vi "히로미사_TEST_2.vi"() -> ()   [LabVIEW 2023]
uses:
  <vilib>/Analysis/3filter.llb/Filter Passband Type.ctl
  <vilib>/Analysis/3filter.llb/Butterworth Filter (DBL).vi
  <vilib>/Analysis/2dsp.llb/1D Cross Correlation (DBL).vi
  <vilib>/Analysis/NI_AALBase.lvlib
  <vilib>/Analysis/NI_AALPro.lvlib
panel:
  in  "불리언":bool
  out "Phase_CR_CI_aTANT":waveform(dbl)(graph)
  out "Amplitude_CR_CI":waveform(dbl)(graph)
  out "Matched_CR_RESULT_Baseband":waveform(dbl)(graph)
  out "Matched_CI_RESULT_Baseband":waveform(dbl)(graph)
  out "Filter_Result_SIN":waveform(dbl)(graph)
  out "Filter_Result_COS":waveform(dbl)(graph)
  out "Local_Result_COS":waveform(dbl)(graph)
  out "Local_Result_SIN":waveform(dbl)(graph)
  out "Matched_CR_Result":waveform(dbl)(graph)
  out "Matched_CI_Result":waveform(dbl)(graph)
  out "RX SIG 그래프":waveform(dbl)(graph)
  in  "Delta_Phase":dbl=90.0 format="%#_13g"
  in  "INIT_phase":dbl=90.0 format="%#_13g"
  out "Mask CR 그래프":waveform(dbl)(graph)
  out "Mask CI 그래프":waveform(dbl)(graph)
  out "Cos_Q 결과 그래프":waveform(dbl)(graph)
  out "Sine_Q 결과 그래프":waveform(dbl)(graph)
  in  "Q":dbl=2.0 format="%#_13g"
  in  "위상":dbl format="%#_13g"
  in  "Fs":dbl=20000.0 format="%#_13g"
  in  "주파수":dbl=5.0 format="%#_13g"
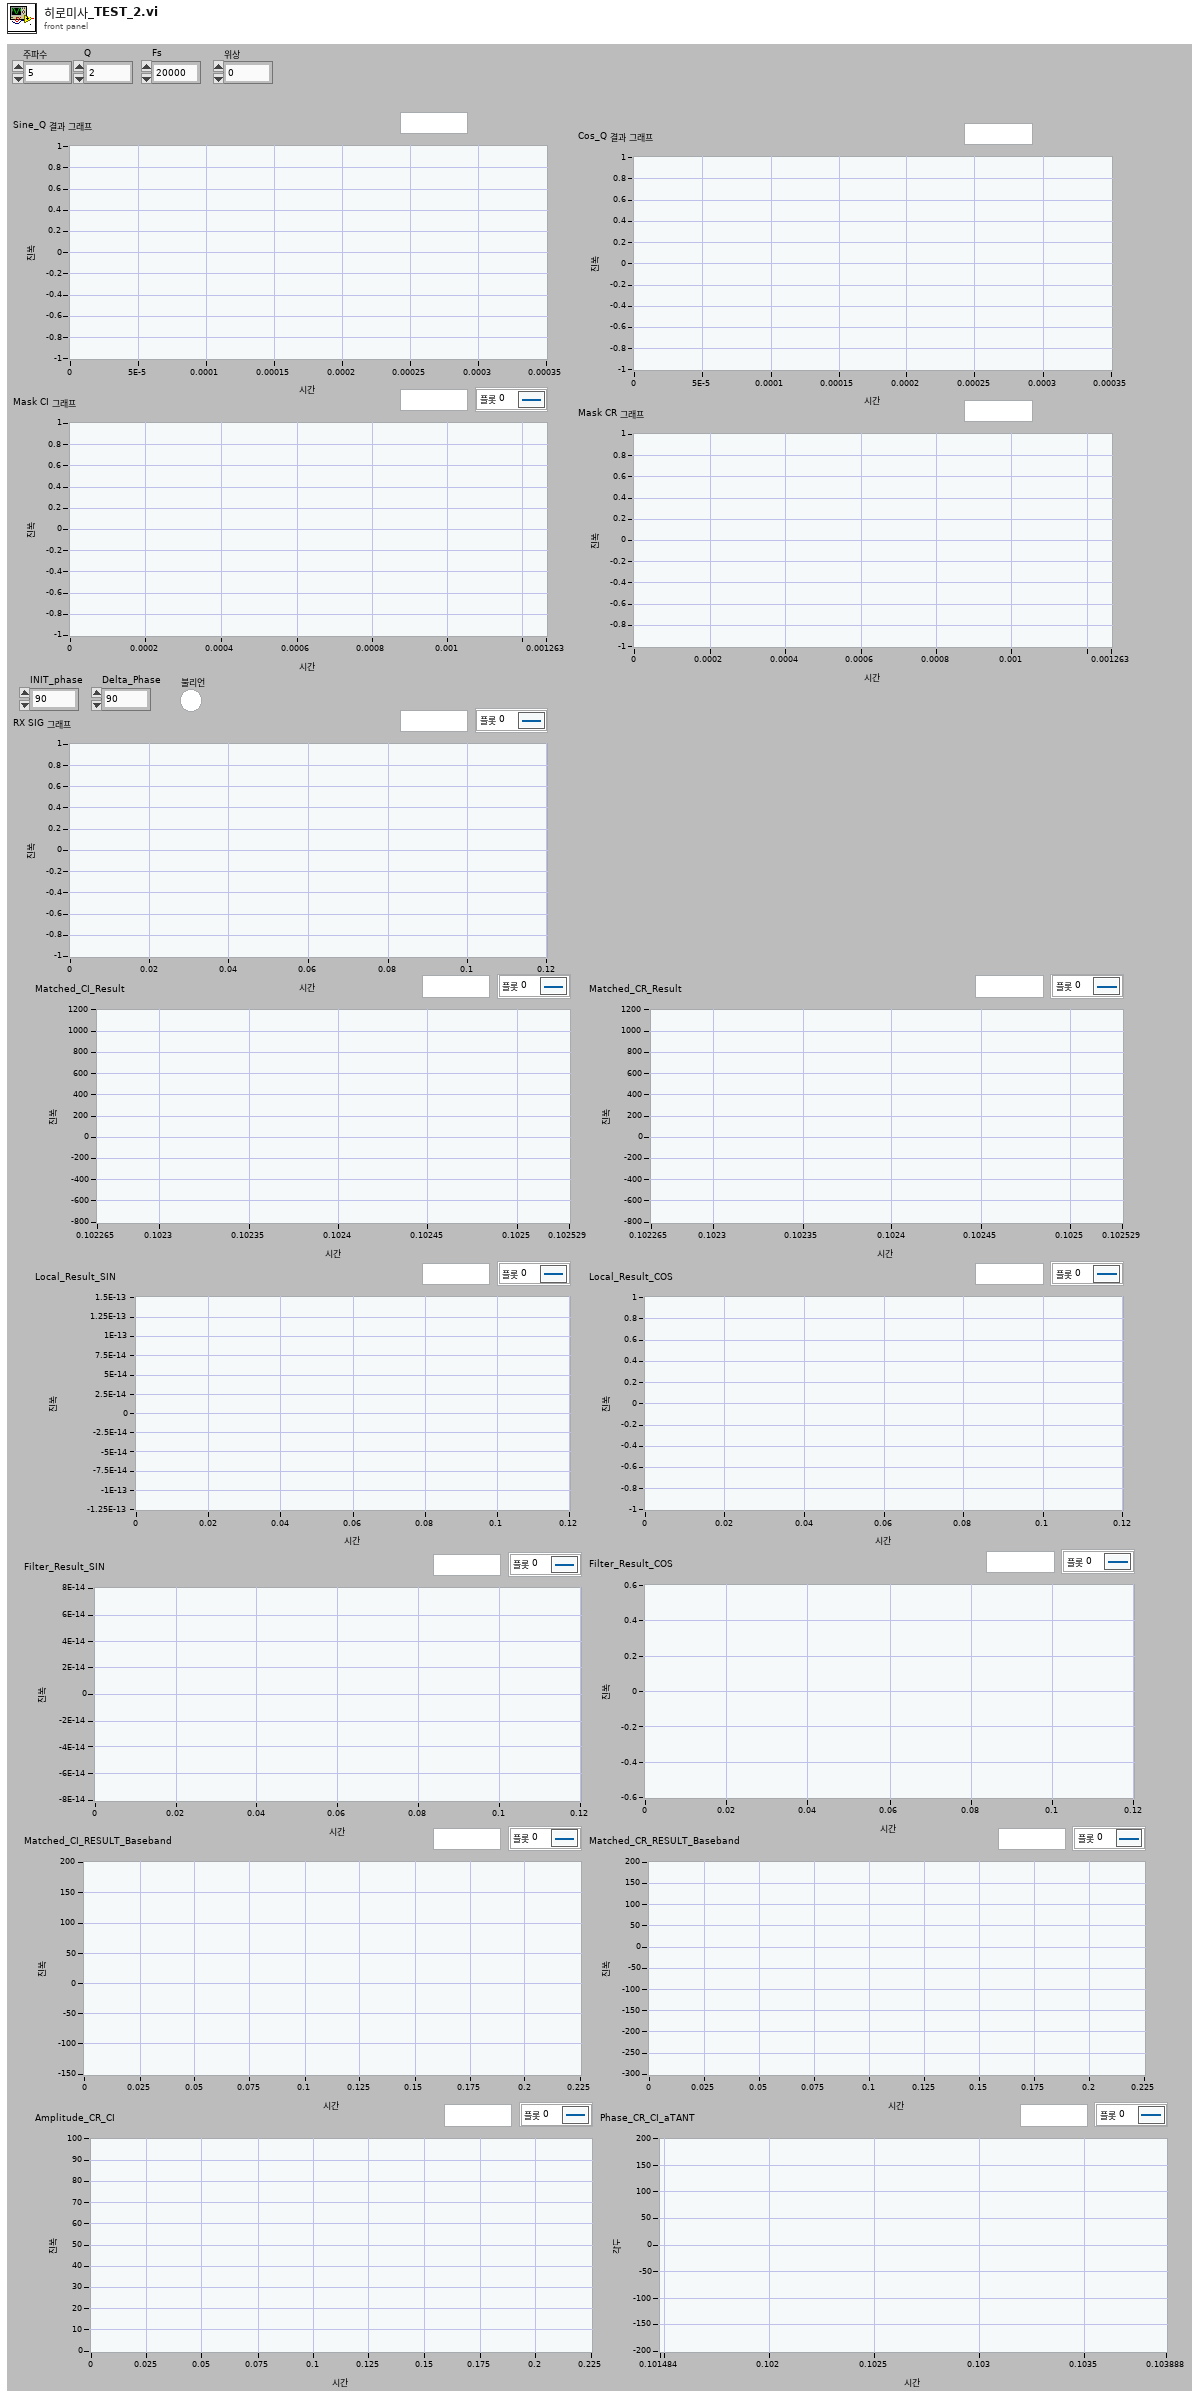
[diagram p1: front panel]
types:
  T1 = typedef "NI_AALBase.lvlib/Filter Passband Type.ctl" = enum32{"Lowpass", "Highpass", "Bandpass", "Bandstop"}
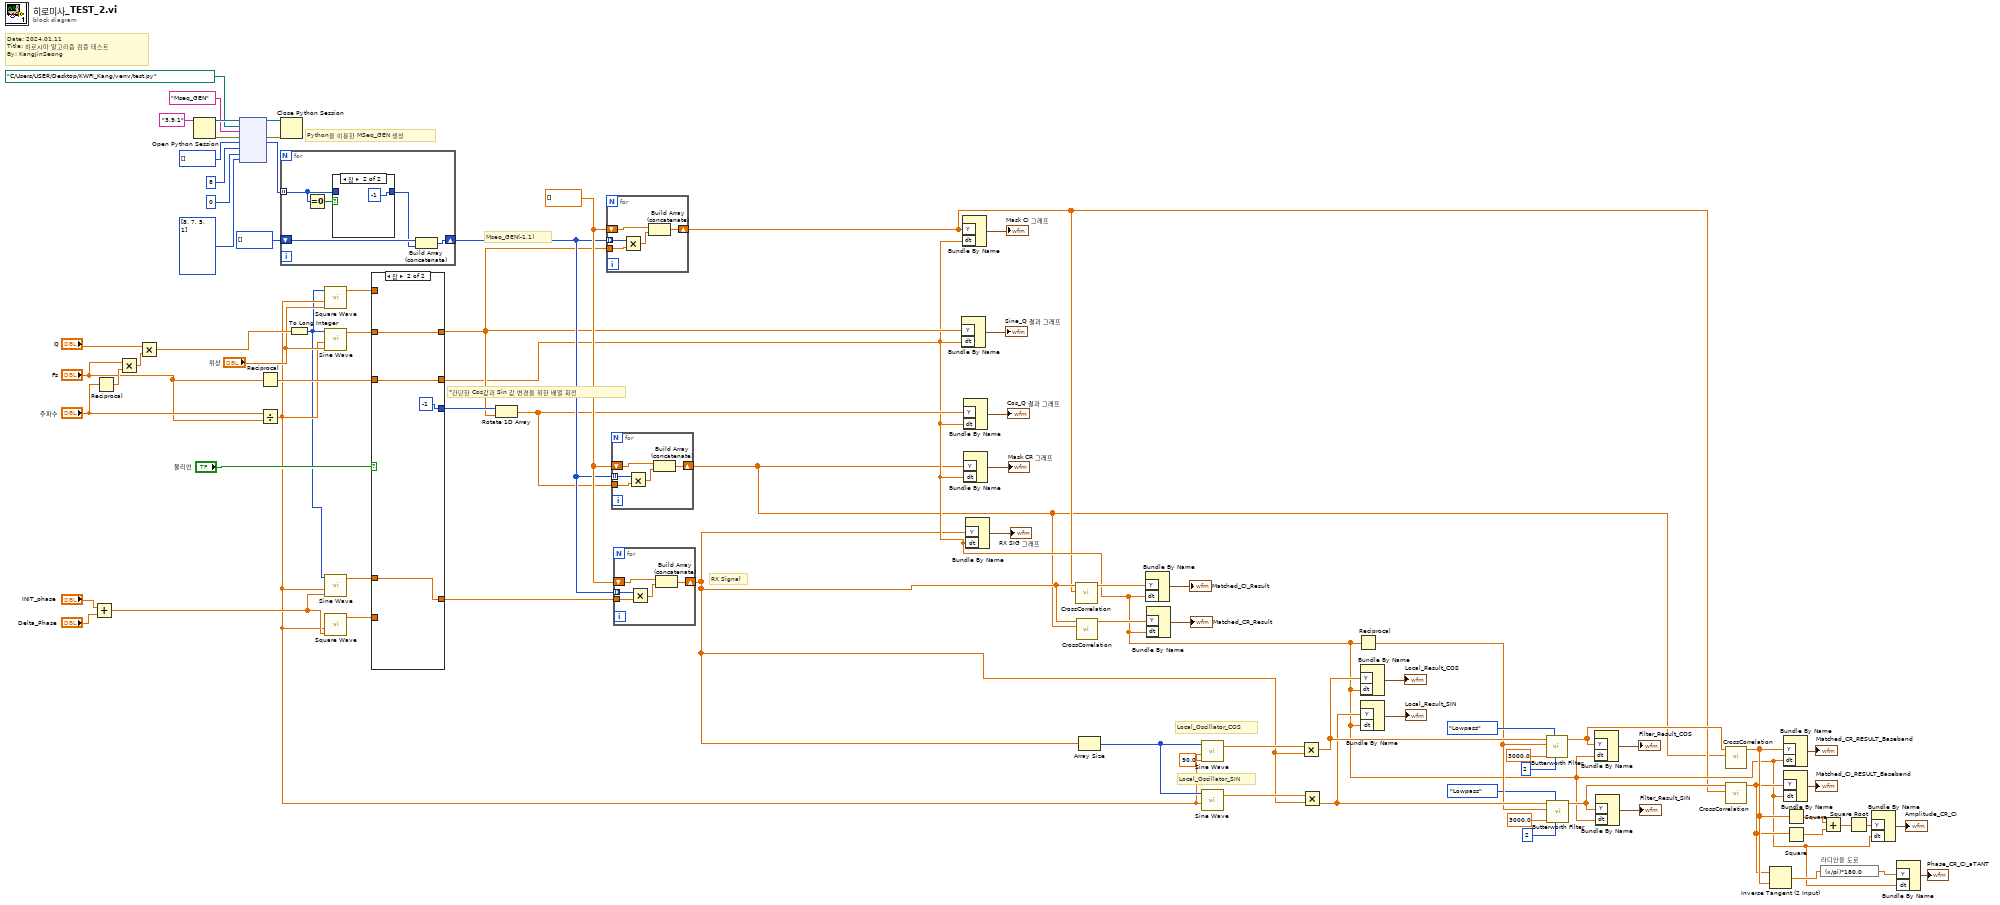
[diagram p0: block diagram]
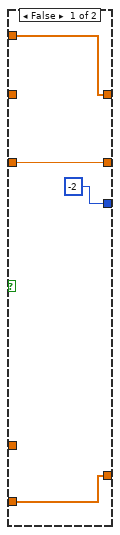
[diagram p2: hidden frame]
diagram:
  w52 = dbl[] []
  # "*간단한 Cos값과 Sin 값 변경을 위한 배열 회전"
  # "Mseq_GEN(-1,1)"
  # "Python을 이용한 MSeq_GEN 생성"
  # "Local_Oscillator_SIN"
  # "Local_Oscillator_COS"
  # "RX Signal"
  # "Date: 2024.01.11\nTitle: 히로시마 알고리즘 검증 테스트\nBy: KangJinSeong"
  n1 = Add(x="INIT_phase", y="Delta_Phase") -> (x+y=w18:dbl)
  n2 = Reciprocal(x="주파수") -> (1/x=w67:dbl)
  n3 = Multiply(x="Fs", y=w67) -> (x*y=w65:dbl)
  n4 = Multiply(x="Q", y=w65) -> (x*y=w63:dbl)
  n5 = Open Python Session(python version="3.9.1" ("Python 버전")) -> (session out=w80:refnum<k35>, error out=w79:errorcluster)  [unwired: 2 in]
  n6 = node(w80, path "C:/Users/USER/Desktop/KWFI_Kang/venv/test.py" ("Python 경로"), "Mseq_GEN" ("함수 이름"), w79, i32[] [], 8, 0, i32[] [8, 7, 5, 1]) -> (w77:refnum<k35>, w78:errorcluster, w69:i32[])  [unwired: 3 in, 2 out]
  n7 = Reciprocal(x="Fs") -> (1/x=w10:dbl)
  n8 = Divide(x="주파수", y="Fs") -> (x/y=w2:dbl)
  n9 = Close Python Session(session in=w77, error in=w78) -> ()  [unwired: 1 out]
  n10 = for {
    tunnel: w69 -> [w83] mode=indexing
    shift-right: [w82] -> w33
    shift-left: i32[] [] -> [w85]
    n11 = Equal To 0?(x=w83) -> (x = 0?=w86:bool)
    n12 = case shown="참" w86 {
      tunnel: [w87 -1] -> w84
      tunnel: w83 -> [w87 _]
      frame False {
      }
      frame True {
      }
    }
    n13 = Build Array (concatenate)(w85, w84) -> (w82:i32[])
  }
  n14 = To Long Integer(number=w63) -> (32bit integer=w1:i32)
  n15 = call <vilib>:"Square Wave.vi"("samples"=w1, "frequency"=w2, "phase in"="위상") -> ("square wave"=w16:dbl[])  [unwired: 3 in, 2 out]
  n16 = call <vilib>:"Sine Wave.vi"("samples"=w1, "frequency"=w2, "phase in"="위상") -> ("sine wave"=w15:dbl[])  [unwired: 2 in, 2 out]
  n17 = call <vilib>:"Sine Wave.vi"("samples"=w1, "frequency"=w2, "phase in"=w18) -> ("sine wave"=w14:dbl[])  [unwired: 2 in, 2 out]
  n18 = call <vilib>:"Square Wave.vi"("frequency"=w2, "phase in"=w18) -> ("square wave"=w12:dbl[])  [unwired: 4 in, 2 out]
  n19 = case shown="참" "불리언" {
    tunnel: w16 -> [w92 _]
    tunnel: w15 -> [_ w96]
    tunnel: [w92 w96] -> w9
    tunnel: w14 -> [_ w95]
    tunnel: [w91 w95] -> w13
    tunnel: w12 -> [w91 _]
    tunnel: [-2 ("n") -1 ("n")] -> w11
    tunnel: w10 -> [w89 w93]
    tunnel: [w89 w93] -> w7
    frame False {
    }
    frame True {
    }
  }
  n20 = Rotate 1D Array(1:w9, 2:w11) -> (0:w8:dbl[])
  n21 = for {
    tunnel: w9 -> [w100]
    tunnel: w33 -> [w101] mode=indexing
    shift-right: [w97] -> w5
    shift-left: w52 -> [w99]
    n22 = Multiply(x=w101, y=w100) -> (x*y=w98:dbl[])
    n23 = Build Array (concatenate)(w99, w98) -> (w97:dbl[])
  }
  n24 = for {
    tunnel: w8 -> [w105]
    tunnel: w33 -> [w106] mode=indexing
    shift-right: [w102] -> w4
    shift-left: w52 -> [w104]
    n25 = Multiply(x=w106, y=w105) -> (x*y=w103:dbl[])
    n26 = Build Array (concatenate)(w104, w103) -> (w102:dbl[])
  }
  n27 = for {
    tunnel: w33 -> [w111] mode=indexing
    shift-right: [w108] -> w6
    shift-left: w52 -> [w110]
    tunnel: w13 -> [w107]
    n28 = Multiply(x=w111, y=w107) -> (x*y=w109:dbl[])
    n29 = Build Array (concatenate)(w110, w109) -> (w108:dbl[])
  }
  n30 = Bundle By Name("Y"=w9, "dt"=w7) -> (→"Sine_Q 결과 그래프":waveform(dbl))  [unwired: 1 in]
  n31 = Bundle By Name("Y"=w5, "dt"=w7) -> (→"Mask CI 그래프":waveform(dbl))  [unwired: 1 in]
  n32 = Bundle By Name("Y"=w8, "dt"=w7) -> (→"Cos_Q 결과 그래프":waveform(dbl))  [unwired: 1 in]
  n33 = Bundle By Name("Y"=w4, "dt"=w7) -> (→"Mask CR 그래프":waveform(dbl))  [unwired: 1 in]
  n34 = Bundle By Name("Y"=w6, "dt"=w7) -> (→"RX SIG 그래프":waveform(dbl))  [unwired: 1 in]
  n35 = call-poly <vilib>:"CrossCorrelation.vi"("Y"=w5, "X"=w6) -> ("Rxy"=w56:dbl[])  [unwired: 8 in, 1 out]
  n36 = call-poly <vilib>:"CrossCorrelation.vi"("Y"=w4, "X"=w6) -> ("Rxy"=w53:dbl[])  [unwired: 8 in, 1 out]
  n37 = Array Size(array=w6) -> (size(s)=w50:i32)
  n38 = Bundle By Name("Y"=w56, "dt"=w7) -> (→"Matched_CI_Result":waveform(dbl))  [unwired: 1 in]
  n39 = Bundle By Name("Y"=w53, "dt"=w7) -> (→"Matched_CR_Result":waveform(dbl))  [unwired: 1 in]
  n40 = call <vilib>:"Sine Wave.vi"("samples"=w50, "frequency"=w2, "phase in"=90.0) -> ("sine wave"=w49:dbl[])  [unwired: 2 in, 2 out]
  n41 = call <vilib>:"Sine Wave.vi"("samples"=w50, "frequency"=w2) -> ("sine wave"=w48:dbl[])  [unwired: 3 in, 2 out]
  n42 = Multiply(x=w49, y=w6) -> (x*y=w45:dbl[])
  n43 = Multiply(x=w48, y=w6) -> (x*y=w38:dbl[])
  n44 = Reciprocal(x=w7) -> (1/x=w36:dbl)
  n45 = Bundle By Name("Y"=w45, "dt"=w7) -> (→"Local_Result_COS":waveform(dbl))  [unwired: 1 in]
  n46 = Bundle By Name("Y"=w38, "dt"=w7) -> (→"Local_Result_SIN":waveform(dbl))  [unwired: 1 in]
  n47 = call-poly <vilib>:"Butterworth Filter.vi"("order"=2, "filter type"=Filter_Passband_Type."Lowpass", "low cutoff freq: fl"=3000.0, "sampling freq: fs"=w36, "X"=w45) -> ("Filtered X"=w35:dbl[])  [unwired: 3 in, 1 out]
  n48 = call-poly <vilib>:"Butterworth Filter.vi"("order"=2, "filter type"=Filter_Passband_Type."Lowpass", "low cutoff freq: fl"=3000.0, "sampling freq: fs"=w36, "X"=w38) -> ("Filtered X"=w34:dbl[])  [unwired: 3 in, 1 out]
  n49 = Bundle By Name("Y"=w35, "dt"=w7) -> (→"Filter_Result_COS":waveform(dbl))  [unwired: 1 in]
  n50 = Bundle By Name("Y"=w34, "dt"=w7) -> (→"Filter_Result_SIN":waveform(dbl))  [unwired: 1 in]
  n51 = call-poly <vilib>:"CrossCorrelation.vi"("Y"=w4, "X"=w35) -> ("Rxy"=w24:dbl[])  [unwired: 8 in, 1 out]
  n52 = call-poly <vilib>:"CrossCorrelation.vi"("Y"=w5, "X"=w34) -> ("Rxy"=w23:dbl[])  [unwired: 8 in, 1 out]
  n53 = Inverse Tangent (2 Input)(1:w24, 2:w23) -> (0:w22:dbl[])
  n54 = Bundle By Name("Y"=w24, "dt"=w7) -> (→"Matched_CR_RESULT_Baseband":waveform(dbl))  [unwired: 1 in]
  n55 = Bundle By Name("Y"=w23, "dt"=w7) -> (→"Matched_CI_RESULT_Baseband":waveform(dbl))  [unwired: 1 in]
  n56 = Square(x=w24) -> (x^2=w30:dbl[])
  n57 = Square(x=w23) -> (x^2=w29:dbl[])
  n58 = expression code="(x/pi)*180.0" "라디안을 도로"(w22) -> (w21:dbl[])
  n59 = Add(x=w30, y=w29) -> (x+y=w28:dbl[])
  n60 = Square Root(x=w28) -> (sqrt(x)=w26:dbl[])
  n61 = Bundle By Name("Y"=w26, "dt"=w7) -> (→"Amplitude_CR_CI":waveform(dbl))  [unwired: 1 in]
  n62 = Bundle By Name("Y"=w21, "dt"=w7) -> (→"Phase_CR_CI_aTANT":waveform(dbl))  [unwired: 1 in]
